vi "new_cheval.vi"(8 "Abort":bool, 9 "Arm Down":bool, 10 "Arm Up":bool, 11 "Start Cheval de Frise":bool) -> (1 "Done":bool, 2 "Arcade Drive":cluster{"x":dbl, "y":dbl}, 3 "Arm Solenoid":bool)   [LabVIEW 2015]
uses:
  new_cheval_state.ctl
  Sensors.vi
panel:
  in  "Kd":dbl format="%#_13g"
  in  "Ki":dbl format="%#_13g"
  in  "Kp":dbl format="%#_13g"
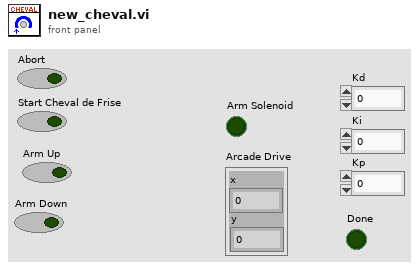
[diagram p1: front panel]
types:
  T1 = typedef "new_cheval_state.ctl" = enum16{"Ready", "Arm Down", "Drive Over", "Arm Up", "Complete"}
  T2 = enum16{"Ready", "Arm Down", "Drive Over", "Arm Up", "Complete"}
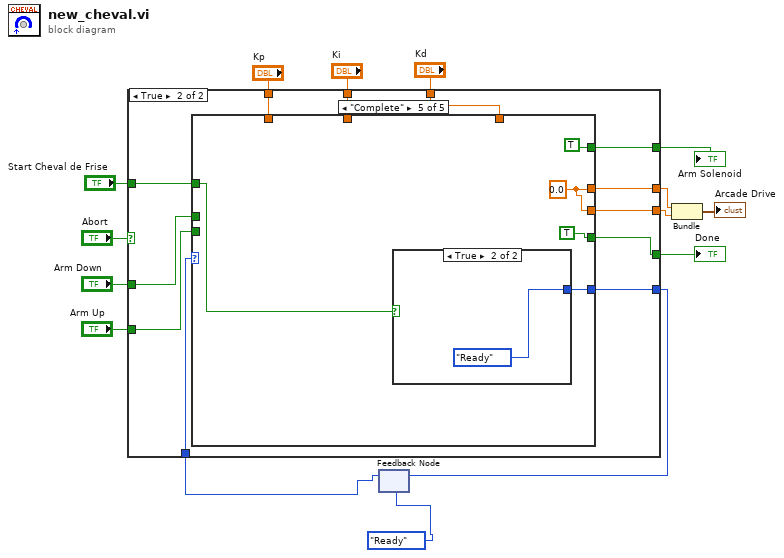
[diagram p0: block diagram]
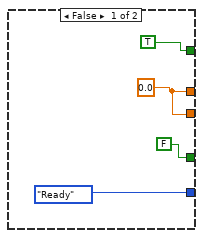
[diagram p2: hidden frame]
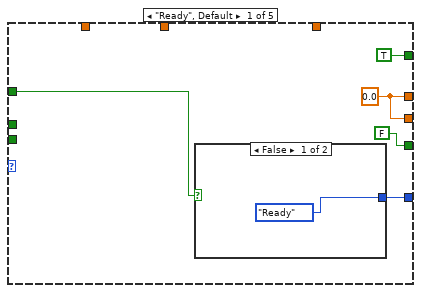
[diagram p3: hidden frame]
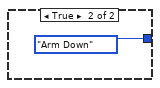
[diagram p4: hidden frame]
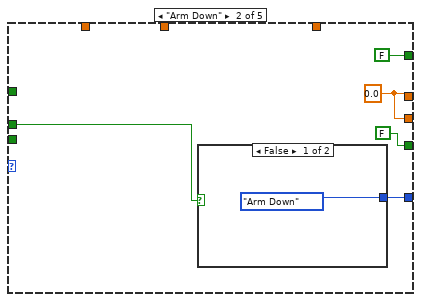
[diagram p5: hidden frame]
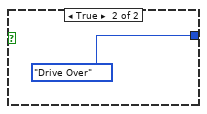
[diagram p6: hidden frame]
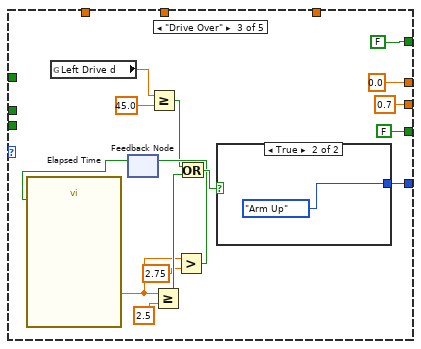
[diagram p7: hidden frame]
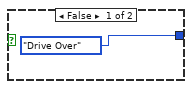
[diagram p8: hidden frame]
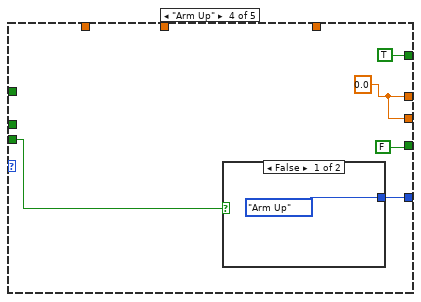
[diagram p9: hidden frame]
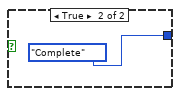
[diagram p10: hidden frame]
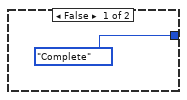
[diagram p11: hidden frame]
diagram:
  n1 = feedback #1(new_cheval_state."Ready") -> (w2:T1)
  n2 = case shown="True" "Abort" {
    tunnel: w2 -> [_ w31]
    tunnel: [T2."Ready" w30] -> w1
    tunnel: [TRUE w29] -> w14
    tunnel: [w19 w28] -> w13
    tunnel: [w19 w27] -> w12
    tunnel: "Start Cheval de Frise" -> [_ w26]
    tunnel: "Arm Down" -> [_ w25]
    tunnel: "Kd" -> [_ w24]
    tunnel: "Ki" -> [_ w23]
    tunnel: "Kp" -> [_ w22]
    tunnel: "Arm Up" -> [_ w21]
    tunnel: [FALSE w20] -> w4
    frame False {
      w19 = 0.0
    }
    frame True {
      n3 = case shown="\"Complete\"" w31 {
        tunnel: [w36 w39 w46 w64 w74] -> w30
        tunnel: [TRUE FALSE FALSE TRUE TRUE] -> w29
        tunnel: [w34 w42 0.0 w63 w73] -> w28
        tunnel: [w34 w42 0.7 ("Drive Thru Speed") w63 w73] -> w27
        tunnel: w26 -> [w33 _ _ _ w71]
        tunnel: w25 -> [_ w41 _ _ _]
        tunnel: w24 -> [_ _ _ _ _]
        tunnel: w23 -> [_ _ _ _ _]
        tunnel: w22 -> [_ _ _ _ _]
        tunnel: w21 -> [_ _ _ w66 _]
        tunnel: [FALSE FALSE FALSE FALSE TRUE] -> w20
        frame "Ready", Default {
          w34 = 0.0
          n4 = case shown="False" w33 {
            tunnel: [new_cheval_state."Ready" new_cheval_state."Arm Down"] -> w36
            frame False {
            }
            frame True {
            }
          }
        }
        frame "Arm Down" {
          w42 = 0.0
          n5 = case shown="False" w41 {
            tunnel: [new_cheval_state."Arm Down" new_cheval_state."Drive Over"] -> w39
            frame False {
            }
            frame True {
            }
          }
        }
        frame "Drive Over" {
          n6 = global read "Sensors.vi" "Left Drive d"() -> (w49:dbl)
          n7 = feedback #2() -> (w52:bool)  [unwired: 1 in]
          n8 = call "Elapsed Time"("Reset"=w52) -> ("Elapsed Time (s)"=w54:dbl)  [unwired: 11 in, 7 out]
          n9 = Greater Or Equal?(x=w49, y=45.0) -> (x >= y?=w47:bool)
          n10 = Greater Or Equal?(x=w54, y=2.5) -> (x >= y?=w56:bool)
          n11 = Greater?(x=w54, y=2.75) -> (0:w53:bool)
          n12 = feedback-in #2(w53) -> ()
          n13 = Or(x=w47, y=w56) -> (x .or. y?=w58:bool)
          n14 = case shown="True" w58 {
            tunnel: [new_cheval_state."Drive Over" new_cheval_state."Arm Up"] -> w46
            frame False {
            }
            frame True {
            }
          }
        }
        frame "Arm Up" {
          w63 = 0.0
          n15 = case shown="False" w66 {
            tunnel: [new_cheval_state."Arm Up" new_cheval_state."Complete"] -> w64
            frame False {
            }
            frame True {
            }
          }
        }
        frame "Complete" {
          w73 = 0.0
          n16 = case shown="True" w71 {
            tunnel: [new_cheval_state."Complete" new_cheval_state."Ready"] -> w74
            frame False {
            }
            frame True {
            }
          }
        }
      }
    }
  }
  "Arm Solenoid" <- w14
  "Done" <- w4
  n17 = feedback-in #1(w1) -> ()
  n18 = Bundle(w13, "Drive Thru Speed"=w12) -> (→"Arcade Drive":cluster{dbl, "Drive Thru Speed":dbl})  [unwired: 1 in]
